vi "Test Program Logging Write Log.vi"(8 "error in":errorcluster, 10 "text":string="Log Start", 11 "Test Program Log File":T1) -> (0 "error out":errorcluster, 3 "refnum out":refnum<file>)   [LabVIEW 2018, in "Support Library.lvlib"]
uses:
  support/Support Library.lvlib
  support/Command Log VIs/File Path.ctl
  support/Command Log VIs/Command Logging.lvlib
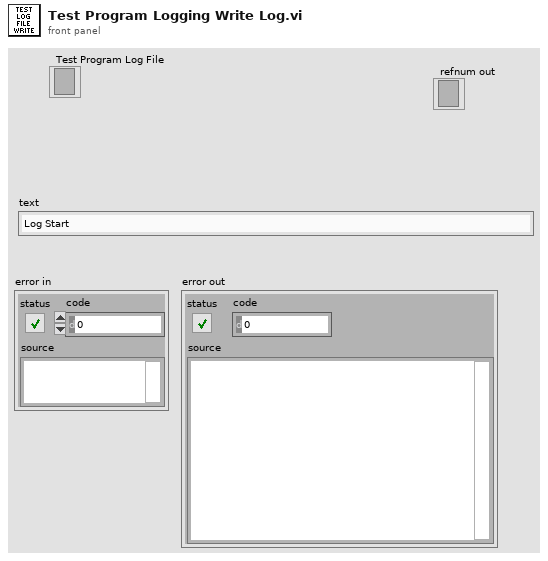
[diagram p1: front panel]
types:
  T1 = typedef "Support Library.lvlib/Command Logging.lvlib/File Path.ctl" = refnum<file>
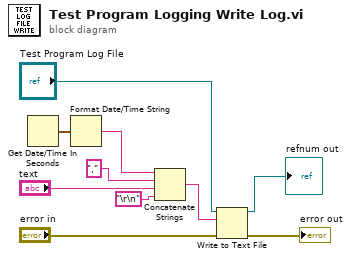
[diagram p0: block diagram]
diagram:
  n1 = Get Date/Time In Seconds() -> (seconds since 1Jan1904=w5:timestamp)
  n2 = Format Date/Time String(seconds (now)=w5) -> (date/time string=w4:string)  [unwired: 2 in]
  n3 = Concatenate Strings(w4, "," ("string"), "text", "\r\n") -> (w8:string)
  n4 = Write to Text File(file (use dialog)="Test Program Log File", text=w8, error in="error in") -> (refnum out=→"refnum out":refnum<file>, error out=→"error out":errorcluster)  [unwired: 1 in, 1 out]
